vi "std.vi"(0 "X":dbl[](array[numeric]) format="%0.2f", 1 "Weighting (Sample)":enum16{"Sample", "Population"}(ring)) -> (2 "mean":dbl format="%0.2f", 3 "Standard Deviation":dbl format="%0.2f", 4 "Variance":dbl format="%0.2f")   [LabVIEW 2020]
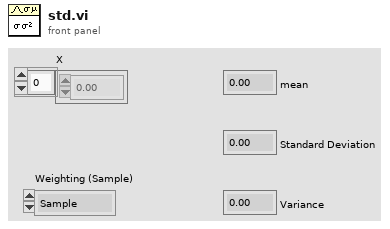
[diagram p1: front panel]
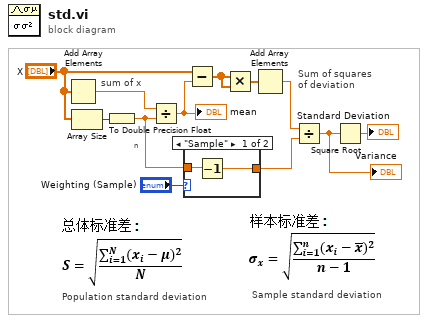
[diagram p0: block diagram]
diagram:
  # "Sum of squares of deviation"
  # "sum of x"
  # "n"
  # "Population standard deviation"
  # "Sample standard deviation"
  n1 = Add Array Elements(numeric array="X") -> (sum=w10:dbl)
  n2 = Array Size(array="X") -> (size(s)=w9:i32)
  n3 = To Double Precision Float(number=w9) -> (double precision float=w8:dbl)
  n4 = Divide(x=w10, y=w8) -> (x/y=w6:dbl)
  "mean" <- w6
  n5 = case shown="\"Sample\"" "Weighting (Sample)" {
    tunnel: w8 -> [w14 w15]
    tunnel: [w13 w15] -> w11
    frame "Sample" {
      n6 = Decrement(x=w14) -> (x-1=w13:dbl)
    }
    frame "Population" {
    }
  }
  n7 = Subtract(x="X", y=w6) -> (x-y=w2:dbl[])
  n8 = Multiply(x=w2, y=w2) -> (x*y=w1:dbl[])
  n9 = Add Array Elements(numeric array=w1) -> (sum=w3:dbl)
  n10 = Divide(x=w3, y=w11) -> (x/y=w4:dbl)
  "Variance" <- w4
  n11 = Square Root(x=w4) -> (sqrt(x)=→"Standard Deviation":dbl)
